vi "linear_ramp_acc_dec.vi"(5 "decel const (dx/dt)":dbl, 7 "accel const (dx/dt)":dbl, 11 "input":dbl) -> (3 "output":dbl)   [LabVIEW 2014]
panel:
  # "dx is in input units\ndt is in seconds"
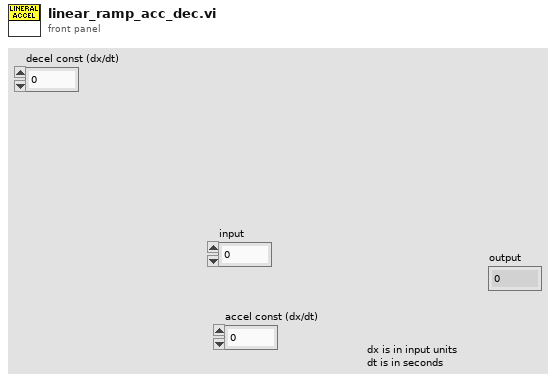
[diagram p1: front panel]
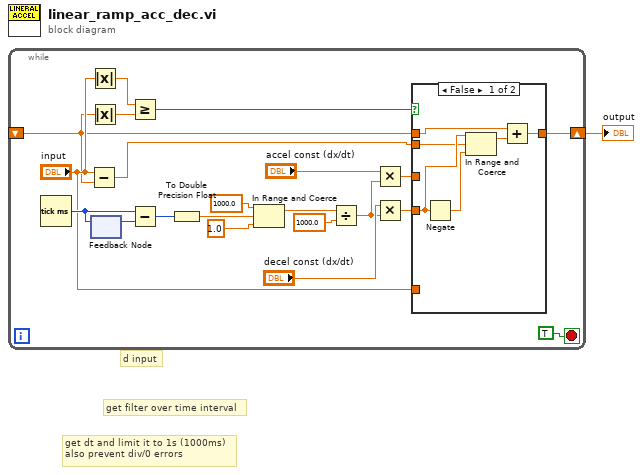
[diagram p0: block diagram]
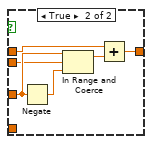
[diagram p2: hidden frame]
diagram:
  # "get filter over time interval"
  # "get dt and limit it to 1s (1000ms)\nalso prevent div/0 errors"
  # "d input"
  n1 = while {
    shift-right: [w12] -> w1
    shift-left: _ -> [w5]
    stop <- TRUE stop-if-true
    n2 = Tick Count (ms)() -> (millisecond timer value=w21:u32)
    n3 = Subtract(x="input", y=w5) -> (x-y=w10:dbl)
    n4 = Absolute Value(x="input") -> (abs(x)=w7:dbl)
    n5 = Absolute Value(x=w5) -> (abs(x)=w8:dbl)
    n6 = feedback-in #1(w21) -> ()
    n7 = feedback #1() -> (w20:u32)  [unwired: 1 in]
    n8 = Greater Or Equal?(x=w7, y=w8) -> (x >= y?=w6:bool)
    n9 = Subtract(x=w21, y=w20) -> (x-y=w19:u32)
    n10 = To Double Precision Float(number=w19) -> (double precision float=w18:dbl)
    n11 = In Range and Coerce(upper limit=1000.0, x=w18, lower limit=1.0) -> (coerced(x)=w14:dbl)  [unwired: 1 out]
    n12 = Divide(x=w14, y=1000.0) -> (x/y=w3:dbl)
    n13 = Multiply(x="accel const (dx/dt)", y=w3) -> (x*y=w11:dbl)
    n14 = Multiply(x="decel const (dx/dt)", y=w3) -> (x*y=w2:dbl)
    n15 = case shown="False" w6 {
      tunnel: [w26 w32] -> w12
      tunnel: w11 -> [_ w31]
      tunnel: w5 -> [w24 w30]
      tunnel: w10 -> [w23 w29]
      tunnel: "input" -> [_ _]
      tunnel: w2 -> [w25 _]
      frame False {
        n16 = Negate(x=w25) -> (-x=w28:dbl)
        n17 = In Range and Coerce(upper limit=w25, x=w23, lower limit=w28) -> (coerced(x)=w27:dbl)  [unwired: 1 out]
        n18 = Add(x=w24, y=w27) -> (x+y=w26:dbl)
      }
      frame True {
        n19 = Negate(x=w31) -> (-x=w34:dbl)
        n20 = In Range and Coerce(upper limit=w31, x=w29, lower limit=w34) -> (coerced(x)=w33:dbl)  [unwired: 1 out]
        n21 = Add(x=w30, y=w33) -> (x+y=w32:dbl)
      }
    }
  }
  "output" <- w1
